vi "Fetch Measurement (Single Sideband Noise).vi"(8 "error in (no error)":errorcluster, 11 "VISA resource name":refnum<visa-resource-name>) -> (0 "error out":errorcluster, 1 "Average SSB Noise (dBm/Hz)":dbl, 2 "Upper or Right SSB Noise (dBm/Hz)":dbl, 3 "VISA resource name out":refnum<visa-resource-name>)   [LabVIEW 2014, in "Agilent ESA PSA Series.lvlib"]
doc: "Returns the results of the last measurement (Single Sideband Noise) and does not initiate data acquisition.\n\n<B>Note:</B>\n\nThis VI is only valid for the Spot Frequency functionality of the Phase noise personality."
uses:
  Agilent ESA PSA Series.lvlib
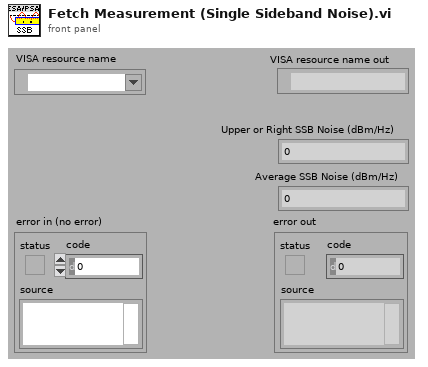
[diagram p1: front panel]
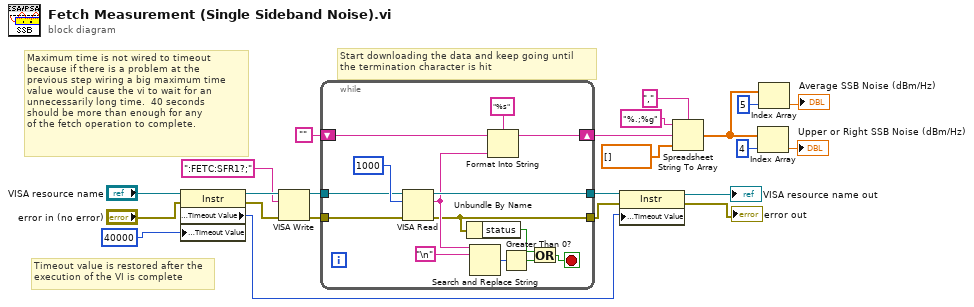
[diagram p0: block diagram]
diagram:
  # "Maximum time is not wired to timeout\nbecause if there is a problem at the\nprevious step wiring a big maximum time\nvalue would cause the vi to wait for an\nunnecessarily long time.  40 seconds\nshould be more than enough for any\nof the fetch operation to complete."
  # "Timeout value is restored after the\nexecution of the VI is complete"
  # "Start downloading the data and keep going until\nthe termination character is hit"
  n1 = property on="Property Node" class="Instr"(reference="VISA resource name", error in="error in (no error)", "General Settings:Timeout Value"=u32 40000) -> (reference out=w4:refnum<visa-resource-name>, error out=w3:errorcluster, "General Settings:Timeout Value"=w19:u32)
  n2 = VISA Write(VISA resource name=w4, write buffer=":FETC:SFR1?;", error in (no error)=w3) -> (VISA resource name out=w6:refnum<visa-resource-name>, error out=w5:errorcluster)  [unwired: 1 out]
  n3 = while {
    tunnel: [w36] -> w21
    tunnel: [w24] -> w20
    tunnel: w6 -> [w35]
    tunnel: w5 -> [w34]
    shift-right: [w30] -> w12
    shift-left: "" -> [w29]
    stop <- w25 stop-if-true
    n4 = VISA Read(VISA resource name=w35, byte count=u32 1000, error in (no error)=w34) -> (VISA resource name out=w36:refnum<visa-resource-name>, read buffer=w31:string, error out=w24:errorcluster)  [unwired: 1 out]
    n5 = Unbundle By Name(w24) -> ("status"=w27:bool)
    n6 = Search and Replace String(input string=w31, search string="\n") -> (number of replacements=w32:i32)  [unwired: 6 in, 3 out]
    n7 = Format Into String(format string="%s", initial string=w29, w31) -> (resulting string=w30:string)  [unwired: 1 in, 1 out]
    n8 = Greater Than 0?(x=w32) -> (x > 0?=w26:bool)
    n9 = Or(x=w27, y=w26) -> (x .or. y?=w25:bool)
  }
  n10 = property on="Property Node" class="Instr"(reference=w21, error in=w20, "General Settings:Timeout Value"=w19) -> (reference out=→"VISA resource name out":refnum<visa-resource-name>, error out=→"error out":errorcluster)
  n11 = Spreadsheet String To Array(delimiter (Tab)=",", format string="%.;%g", spreadsheet string=w12, array type (2D Dbl)=dbl[] []) -> (array=w10:dbl[])
  n12 = Index Array(array=w10, index=4) -> (element=→"Upper or Right SSB Noise (dBm/Hz)":dbl)
  n13 = Index Array(array=w10, index=5) -> (element=→"Average SSB Noise (dBm/Hz)":dbl)
